vi "Configure Acquisition.vi"(4 "Reference Signal (0: Off)":i32(ring) items=["Off", "Out", "In"], 5 "Segment Count (2)":i32=2, 6 "Segment Index (1)":i32=1, 7 "Average Count (8)":dbl=8.0, 8 "error in (no error)":errorcluster, 9 "Acquisition Type (0: Normal)":i32(ring) items=["Normal", "Average", "High Resolution", "Peak"], 10 "Acquisition Format (0: Real-time)":i32(ring) items=["Real-time", "Segmented", "Equivalent-time", " Real-time (Max Update Rate)"], 11 "VISA resource name":refnum<visa-resource-name>) -> (0 "error out":errorcluster, 3 "VISA resource name out":refnum<visa-resource-name>)   [LabVIEW 2015, in "Agilent 2000 3000 X-Series.lvlib"]
doc: "Configure the acquisition settings."
uses:
  Agilent 2000 3000 X-Series.lvlib
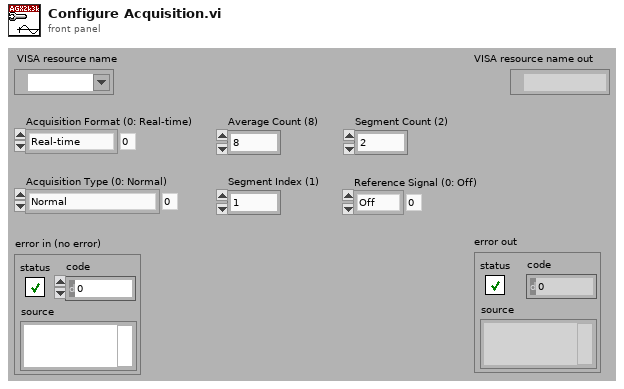
[diagram p1: front panel]
types:
  T1 = typedef "Agilent 2000 3000 X-Series.lvlib/Extended User Data.ctl" = cluster{"X-Series Mode":u16, "Acquisition Type (0: Normal)":i32}
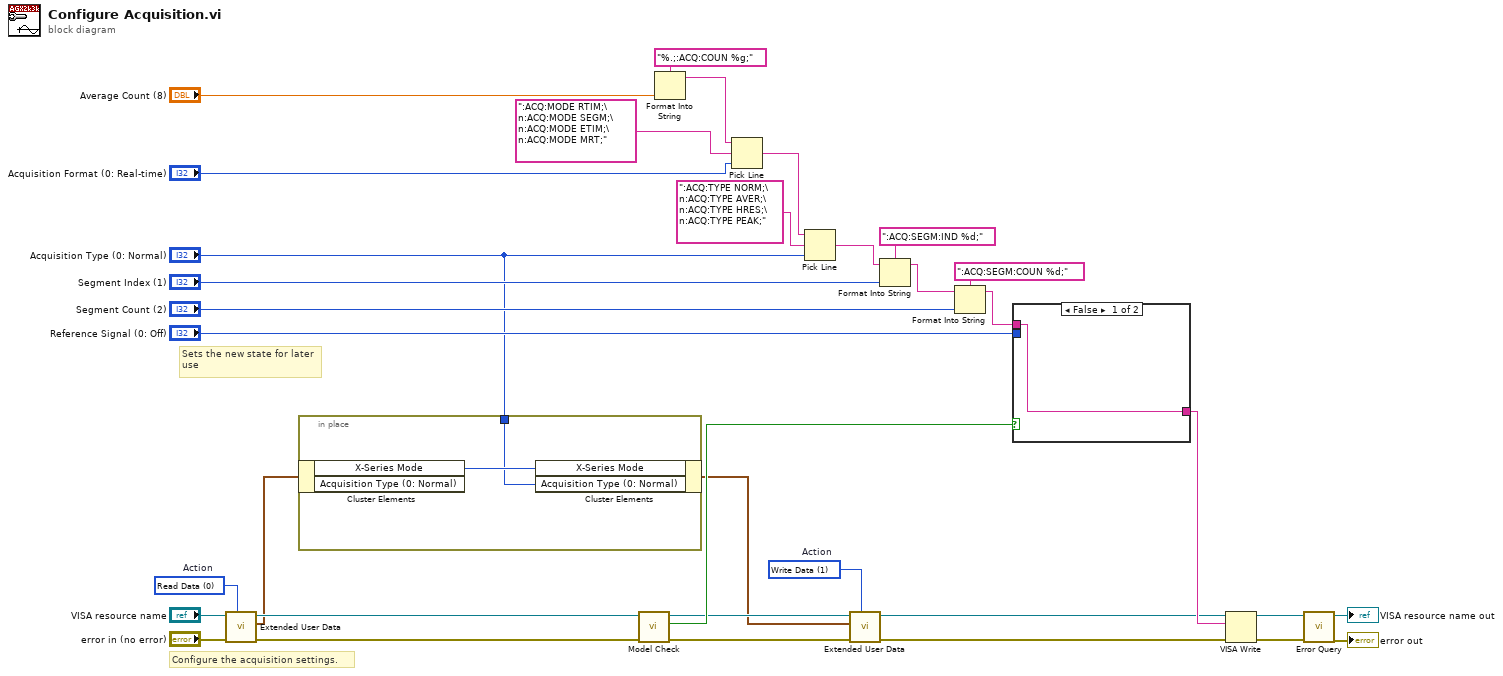
[diagram p0: block diagram]
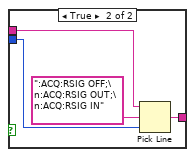
[diagram p2: hidden frame]
diagram:
  w4 = 1 items=["Read Data", "Write Data", "Clear Data", "Clear ALL Data"]  # Action
  w5 = 0 items=["Read Data", "Write Data", "Clear Data", "Clear ALL Data"]  # Action
  # "Sets the new state for later\nuse"
  # "Configure the acquisition settings."
  n1 = call "Extended User Data.vi"("Action (1: Write Data)"=w5, "error in (no error)"="error in (no error)", "VISA resource name in"="VISA resource name") -> ("error out"=w9:errorcluster, "User Data Out"=w3:T1, "VISA resource name out"=w8:refnum<visa-resource-name>)  [unwired: 6 in]
  n2 = in-place {
    in-place-border: "Acquisition Type (0: Normal)" -> [w35]
    n3 = in-place-cluster #1(w3) -> ("X-Series Mode"=w36:u16)  [unwired: 1 out]
    n4 = in-place-cluster #1("X-Series Mode"=w36, "Acquisition Type (0: Normal)"=w35) -> (w1:T1)
  }
  n5 = call "Model Check.vi"("error in (no error)"=w9, "VISA resource name"=w8) -> ("error out"=w13:errorcluster, "Not 2000 or 3000 Series"=w14:bool, "VISA resource name out"=w12:refnum<visa-resource-name>)  [unwired: 7 out]
  n6 = Format Into String(format string="%.;:ACQ:COUN %g;", "Average Count (8)") -> (resulting string=w30:string)  [unwired: 2 in, 1 out]
  n7 = Pick Line(string ("")=w30, multi-line string=":ACQ:MODE RTIM;\n:ACQ:MODE SEGM;\n:ACQ:MODE ETIM;\n:ACQ:MODE MRT;", line index="Acquisition Format (0: Real-time)") -> (output string=w28:string)
  n8 = Pick Line(string ("")=w28, multi-line string=":ACQ:TYPE NORM;\n:ACQ:TYPE AVER;\n:ACQ:TYPE HRES;\n:ACQ:TYPE PEAK;", line index="Acquisition Type (0: Normal)") -> (output string=w27:string)
  n9 = call "Extended User Data.vi"("Action (1: Write Data)"=w4, "error in (no error)"=w13, "User Data In"=w1, "VISA resource name in"=w12) -> ("error out"=w10:errorcluster, "VISA resource name out"=w11:refnum<visa-resource-name>)  [unwired: 5 in, 1 out]
  n10 = Format Into String(format string=":ACQ:SEGM:IND %d;", initial string=w27, "Segment Index (1)") -> (resulting string=w24:string)  [unwired: 1 in, 1 out]
  n11 = Format Into String(format string=":ACQ:SEGM:COUN %d;", initial string=w24, "Segment Count (2)") -> (resulting string=w17:string)  [unwired: 1 in, 1 out]
  n12 = case shown="False" w14 {
    tunnel: w17 -> [w37 w40]
    tunnel: [w37 w39] -> w15
    tunnel: "Reference Signal (0: Off)" -> [_ w38]
    frame False {
    }
    frame True {
      n13 = Pick Line(string ("")=w40, multi-line string=":ACQ:RSIG OFF;\n:ACQ:RSIG OUT;\n:ACQ:RSIG IN", line index=w38) -> (output string=w39:string)
    }
  }
  n14 = VISA Write(VISA resource name=w11, write buffer=w15, error in (no error)=w10) -> (VISA resource name out=w21:refnum<visa-resource-name>, error out=w20:errorcluster)  [unwired: 1 out]
  n15 = call "Error Query.vi"("error in (no error)"=w20, "VISA resource name"=w21) -> ("error out"=→"error out":errorcluster, "VISA resource name out"=→"VISA resource name out":refnum<visa-resource-name>)  [unwired: 8 out]
